vi "Controller.vi"(0 "x":dbl, 1 "y":dbl, 2 "x_dot":dbl, 3 "y_dot":dbl, 4 "Stiff":dbl, 6 "Damp":dbl) -> (7 "f_x":dbl, 8 "f_y":dbl)   [LabVIEW 2017]
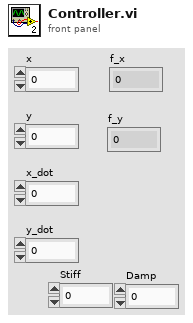
[diagram p1: front panel]
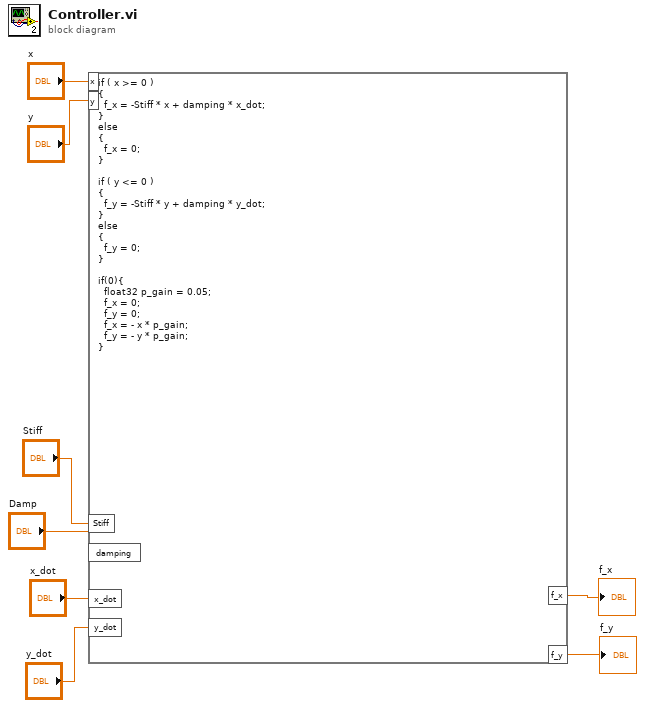
[diagram p0: block diagram]
diagram:
  n1 = formula code="if ( x >= 0 )\n{\n  f_x = -Stiff * x + damping * x_dot;\n}\nelse\n{\n  f_x = 0;\n}\n\nif ( y <= 0 )\n{\n  f_y = -Stiff * y + damping * y_dot;\n}\nelse\n{\n  f_y = 0;\n}\n\nif(0){\n  float32 p_gain = 0.05;\n  f_x = 0;\n  f_y = 0;\n  f_x = - x * p_gain;\n  f_y = - y * p_gain;\n}"("x"="x", "y"="y", "x_dot"="x_dot", "y_dot"="y_dot", "Stiff"="Stiff", "damping"="Damp") -> ("f_x"=→"f_x":dbl, "f_y"=→"f_y":dbl)
